vi "Open IPS.vi"(8 "error in (no error)":errorcluster, 11 "Instrument.OxfordVRM in":refnum<class "Instrument.OxfordVRM.lvclass">) -> (0 "error out":errorcluster, 3 "Instrument.OxfordVRM out":refnum<class "Instrument.OxfordVRM.lvclass">)   [LabVIEW 2019, in "Instrument.OxfordVRM.lvclass"]
uses:
  Instrument.OxfordVRM.lvclass
  <instrlib>/Mercury iXX/Public/Controls/Comms Transport Layer.ctl
  Instrument.OxfordVRM.lvclass/Instrument.OxfordVRM.ctl
  <instrlib>/Mercury iXX/Public/Libraries/System/Open/Open System.vi
  <instrlib>/Mercury iXX/Public/Libraries/System/Read/Catalogue (Read).vi
  <instrlib>/Mercury iXX/Mercury iXX.lvlib
  <instrlib>/Mercury iXX/Public/Libraries/System.lvlib
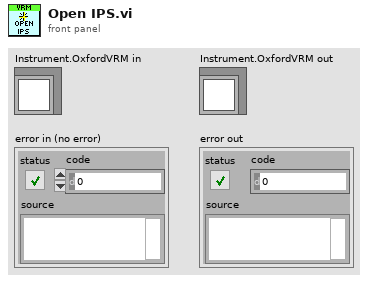
[diagram p1: front panel]
types:
  T1 = typedef "Mercury iXX.lvlib/Comms Transport Layer.ctl" = enum16{"Ethernet TCP/IP", "USB", "ISOBus - RS-232", "GPIB"}
  T2 = typedef "Mercury iXX.lvlib/Mercury Reference.ctl" = cluster{"Comms":refnum<visa-resource-name>, "Device ID":string[], "Comms Layer":T1, "Command":string, "Query reference":T3}
  T3 = typedef "Mercury iXX.lvlib/Query Dynamic Reference.ctl" = refnum<vi>
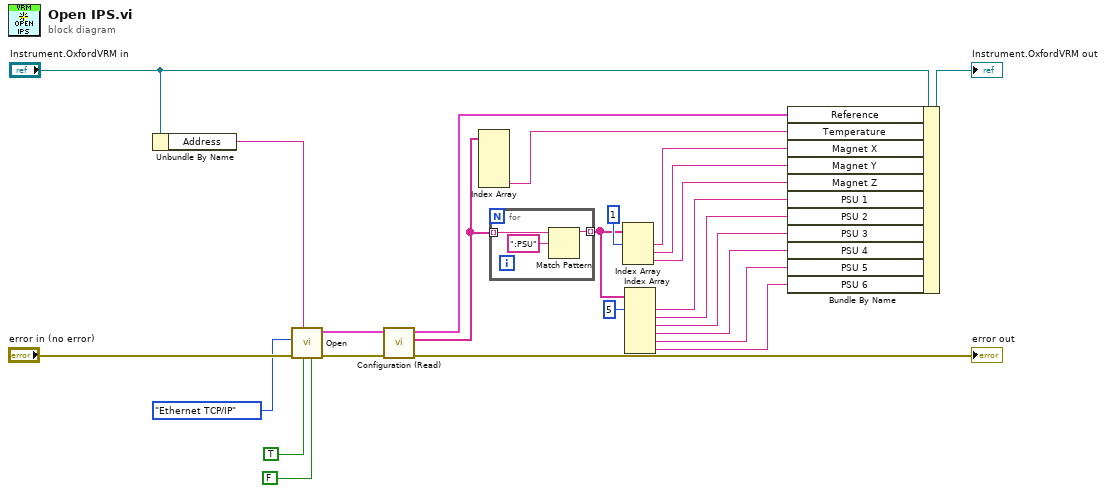
[diagram p0: block diagram]
diagram:
  n1 = Unbundle By Name("Instrument.OxfordVRM in") -> ("Address"=w3:string)
  n2 = call-poly <instrlib>:"Open.vi"("Clear Previous Connections (False)"=FALSE, "ID Query (True)"=TRUE, "IP Address"=w3, "error in (no error)"="error in (no error)", "Comms Layer"=Comms_Transport_Layer."Ethernet TCP/IP") -> ("error out"=w19:errorcluster, "Mercury Reference Out"=w20:T2)  [unwired: 2 in, 3 out]
  n3 = call-poly <instrlib>:"Configuration (Read).vi"("error in"=w19, "Mercury Reference In"=w20) -> ("error out"=→"error out":errorcluster, "Devices"=w23:string[], "Mercury Reference Out"=w21:T2)  [unwired: 1 in, 6 out]
  n4 = Index Array(array=w23) -> (element #5=w15:string)  [unwired: 5 in, 4 out]
  n5 = for {
    tunnel: w23 -> [w27] mode=indexing
    tunnel: [w26] -> w11 mode=indexing
    n6 = Match Pattern(string=w27, regular expression=":PSU") -> (before substring=w26:string)  [unwired: 1 in, 3 out]
  }
  n7 = Index Array(array=w11, index #1=1 ("index")) -> (element #1=w14:string, element #2=w13:string, element #3=w12:string)  [unwired: 2 in]
  n8 = Index Array(array=w11, index #1=5 ("index")) -> (element #1=w9:string, element #2=w8:string, element #3=w7:string, element #4=w6:string, element #5=w5:string, element #6=w4:string)  [unwired: 5 in]
  n9 = Bundle By Name(cluster="Instrument.OxfordVRM in", "Reference"=w21, "Temperature"=w15, "Magnet X"=w14, "Magnet Y"=w13, "Magnet Z"=w12, "PSU 1"=w9, "PSU 2"=w8, "PSU 3"=w7, "PSU 4"=w6, "PSU 5"=w5, "PSU 6"=w4) -> (→"Instrument.OxfordVRM out":refnum<class "Instrument.OxfordVRM.lvclass">)
